vi "twoMPU_alejMarch07.vi"() -> ()   [LabVIEW 2016]
uses:
  <vilib>/MakerHub/LINX/Private/Type Defs/Interface.ctl
  <vilib>/MakerHub/LINX/Public/Sensors/Accelerometer/MPU60X0/Clock Source.ctl
  Control 1.ctl
  <vilib>/MakerHub/LINX/Private/Type Defs/User Platform.ctl
  <vilib>/MakerHub/LINX/Public/Sensors/Accelerometer/MPU60X0/DeviceAddresses.ctl
  <vilib>/MakerHub/LINX/Public/Sensors/Accelerometer/MPU60X0/AccelFullScaleRanges.ctl
  <vilib>/MakerHub/LINX/Public/Sensors/Accelerometer/MPU60X0/GyroFullScaleRanges.ctl
  <vilib>/MakerHub/LINX/Public/Initialize.vi
  <vilib>/express/express shared/transition.llb/Dynamic To Waveform Array.vi
  <vilib>/express/express signal manip/GetorSetDDTAttributes/Set DDT Attributes/SetT0.vi
  <vilib>/express/express shared/transition.llb/Waveform Array To Dynamic.vi
  <vilib>/express/express signal manip/GetorSetDDTAttributes/Set DDT Attributes/Set DDT Properties.xnode
  <vilib>/MakerHub/LINX/LMH-LINX.lvlib
  <vilib>/MakerHub/LINX/Public/Sensors/Accelerometer/MPU60X0/MPU60X0.lvlib
  <vilib>/Platform/NI_3dgraph.lvlib
panel:
  out "Path Length MPU2":dbl
  in  "DATA RECORD":bool
  out "XY Graph 2":cluster{"Y":dbl[], "Y":dbl[]}[](graph)
  in  "Baud Rate Override":T1
  in  "Clock Source 2":T2
  out "Path Length MPU1":dbl
  out "vector error":errorcluster
  in  "Plot of roll and pitch":refnum<k7>(container)
  out "XY Graph":cluster{"Y":dbl[], "Y":dbl[]}[](graph)
  out "error out":errorcluster
  out "MATLAB Error":errorcluster
  out "Error Out":errorcluster
  in  "?":bool
  in  "I2C Channel":u8
  in  "Clock Source":T2
  in  "Interface":T3
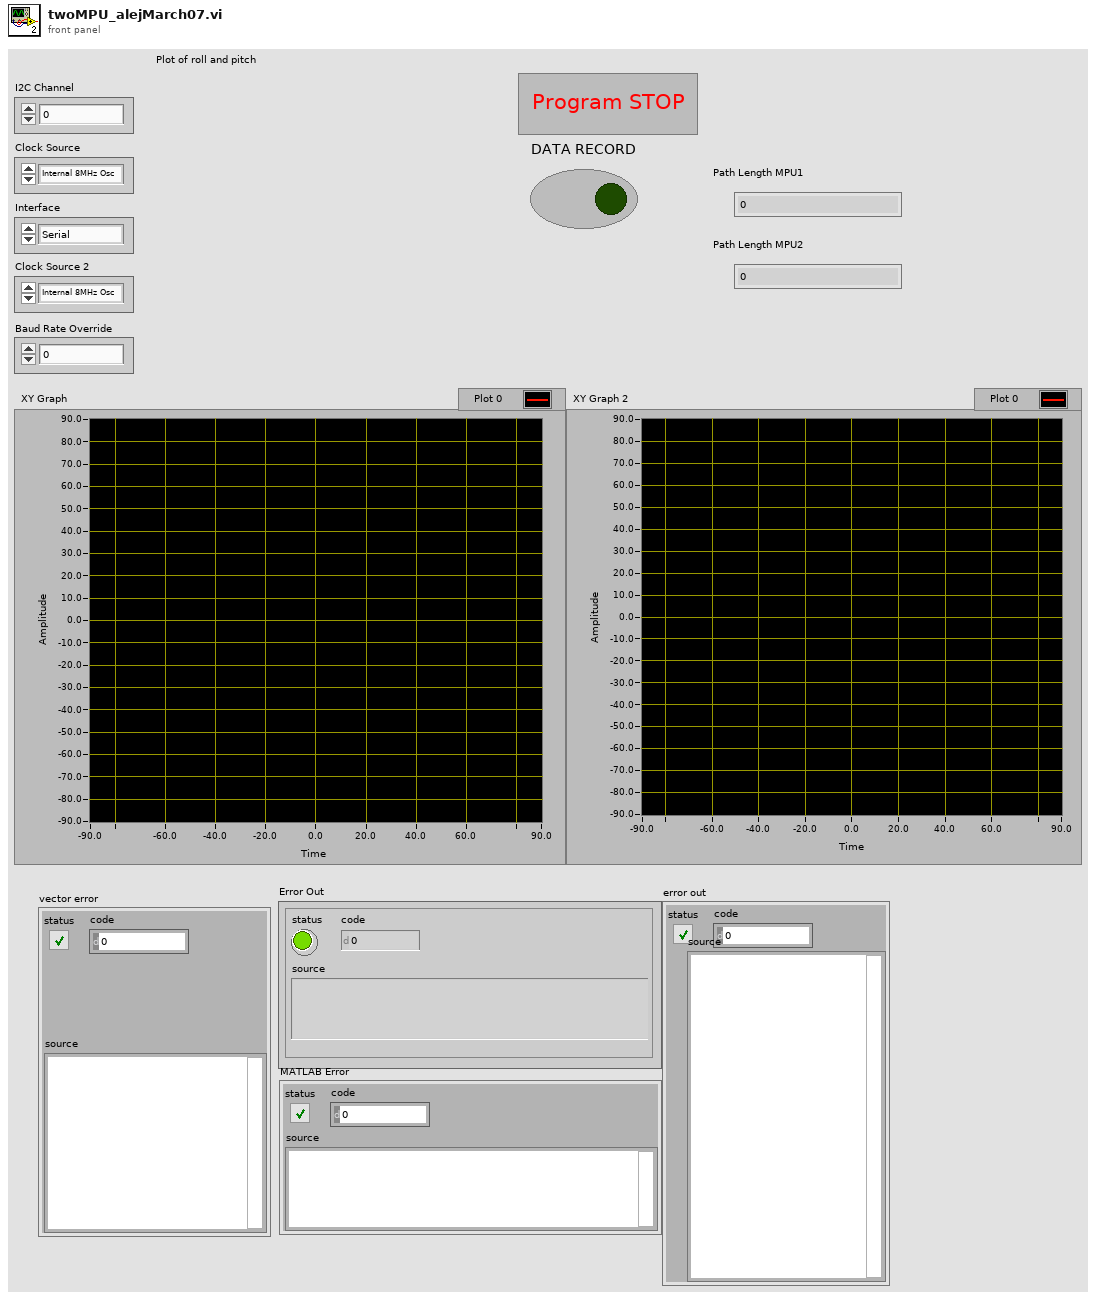
[diagram p1: front panel]
types:
  T1 = typedef "Control 1.ctl" = u32
  T2 = typedef "LMH-LINX.lvlib/MPU60X0.lvlib/Clock Source.ctl" = enum8{"Internal 8MHz Osc", "PLL with X Gyro Ref", "PLL with Y Gyro Ref", "PLL with Z Gyro Ref", "PLL with ext 32.768 KHz Ref", "PLL with ext 19.2 MHz Ref", "Reserved", "Hold in reset"}
  T3 = typedef "LMH-LINX.lvlib/Interface.ctl" = enum16{"Serial", "TCP"}
  T4 = typedef "LMH-LINX.lvlib/MPU60X0.lvlib/DeviceAddresses.ctl" = enum16{"0x68", "0x69"}
  T5 = typedef "LMH-LINX.lvlib/MPU60X0.lvlib/GyroFullScaleRanges.ctl" = enum8{"±250 °/s", "±500 °/s", "±1000 °/s", "±2000 °/s"}
  T6 = typedef "LMH-LINX.lvlib/MPU60X0.lvlib/AccelFullScaleRanges.ctl" = enum16{"±2g", "±4g", "±8g", "±16g"}
  T7 = typedef "LMH-LINX.lvlib/User Platform.ctl" = enum16{"Default", "Remote", "Local"}
  T8 = typedef "LMH-LINX.lvlib/LINX Ref.ctl" = cluster{"IO":T9, "Interface":T3, "LINX Device Config":T10}
  T9 = typedef "LMH-LINX.lvlib/Platform.ctl" = enum16{"Remote", "Local"}
  T10 = typedef "LMH-LINX.lvlib/Device.lvlib/LINX Device Config.ctl" = cluster{"Interface":T3, "COM Port":refnum<visa-resource-name>, "TCP Configuration":T11, "Device Family":u8, "Device ID":u8, "Device Name":string, "TCP Ref":refnum<k5>, "Channels":T12}
  T11 = typedef "LMH-LINX.lvlib/Device.lvlib/TCP Config.ctl" = cluster{"IP Address":string, "Port":u16}
  T12 = typedef "LMH-LINX.lvlib/Channels.ctl" = cluster{"DI":u8[], "DO":u8[], "AI":u8[], "AO":u8[], "PWM":u8[], "QE":u8[], "UART":u8[], "I2C 2":u8[], "SPI":u8[], "CAN":u8[], "Servo":u8[], "AI Ref (V)":dbl, "AI Resolution (Bits)":u8, "AO Ref (V)":dbl, "AO Resolution (Bits)":u8}
  T13 = cluster{"X Axis":i16, "Y Axis":i16, "Z Axis":i16}
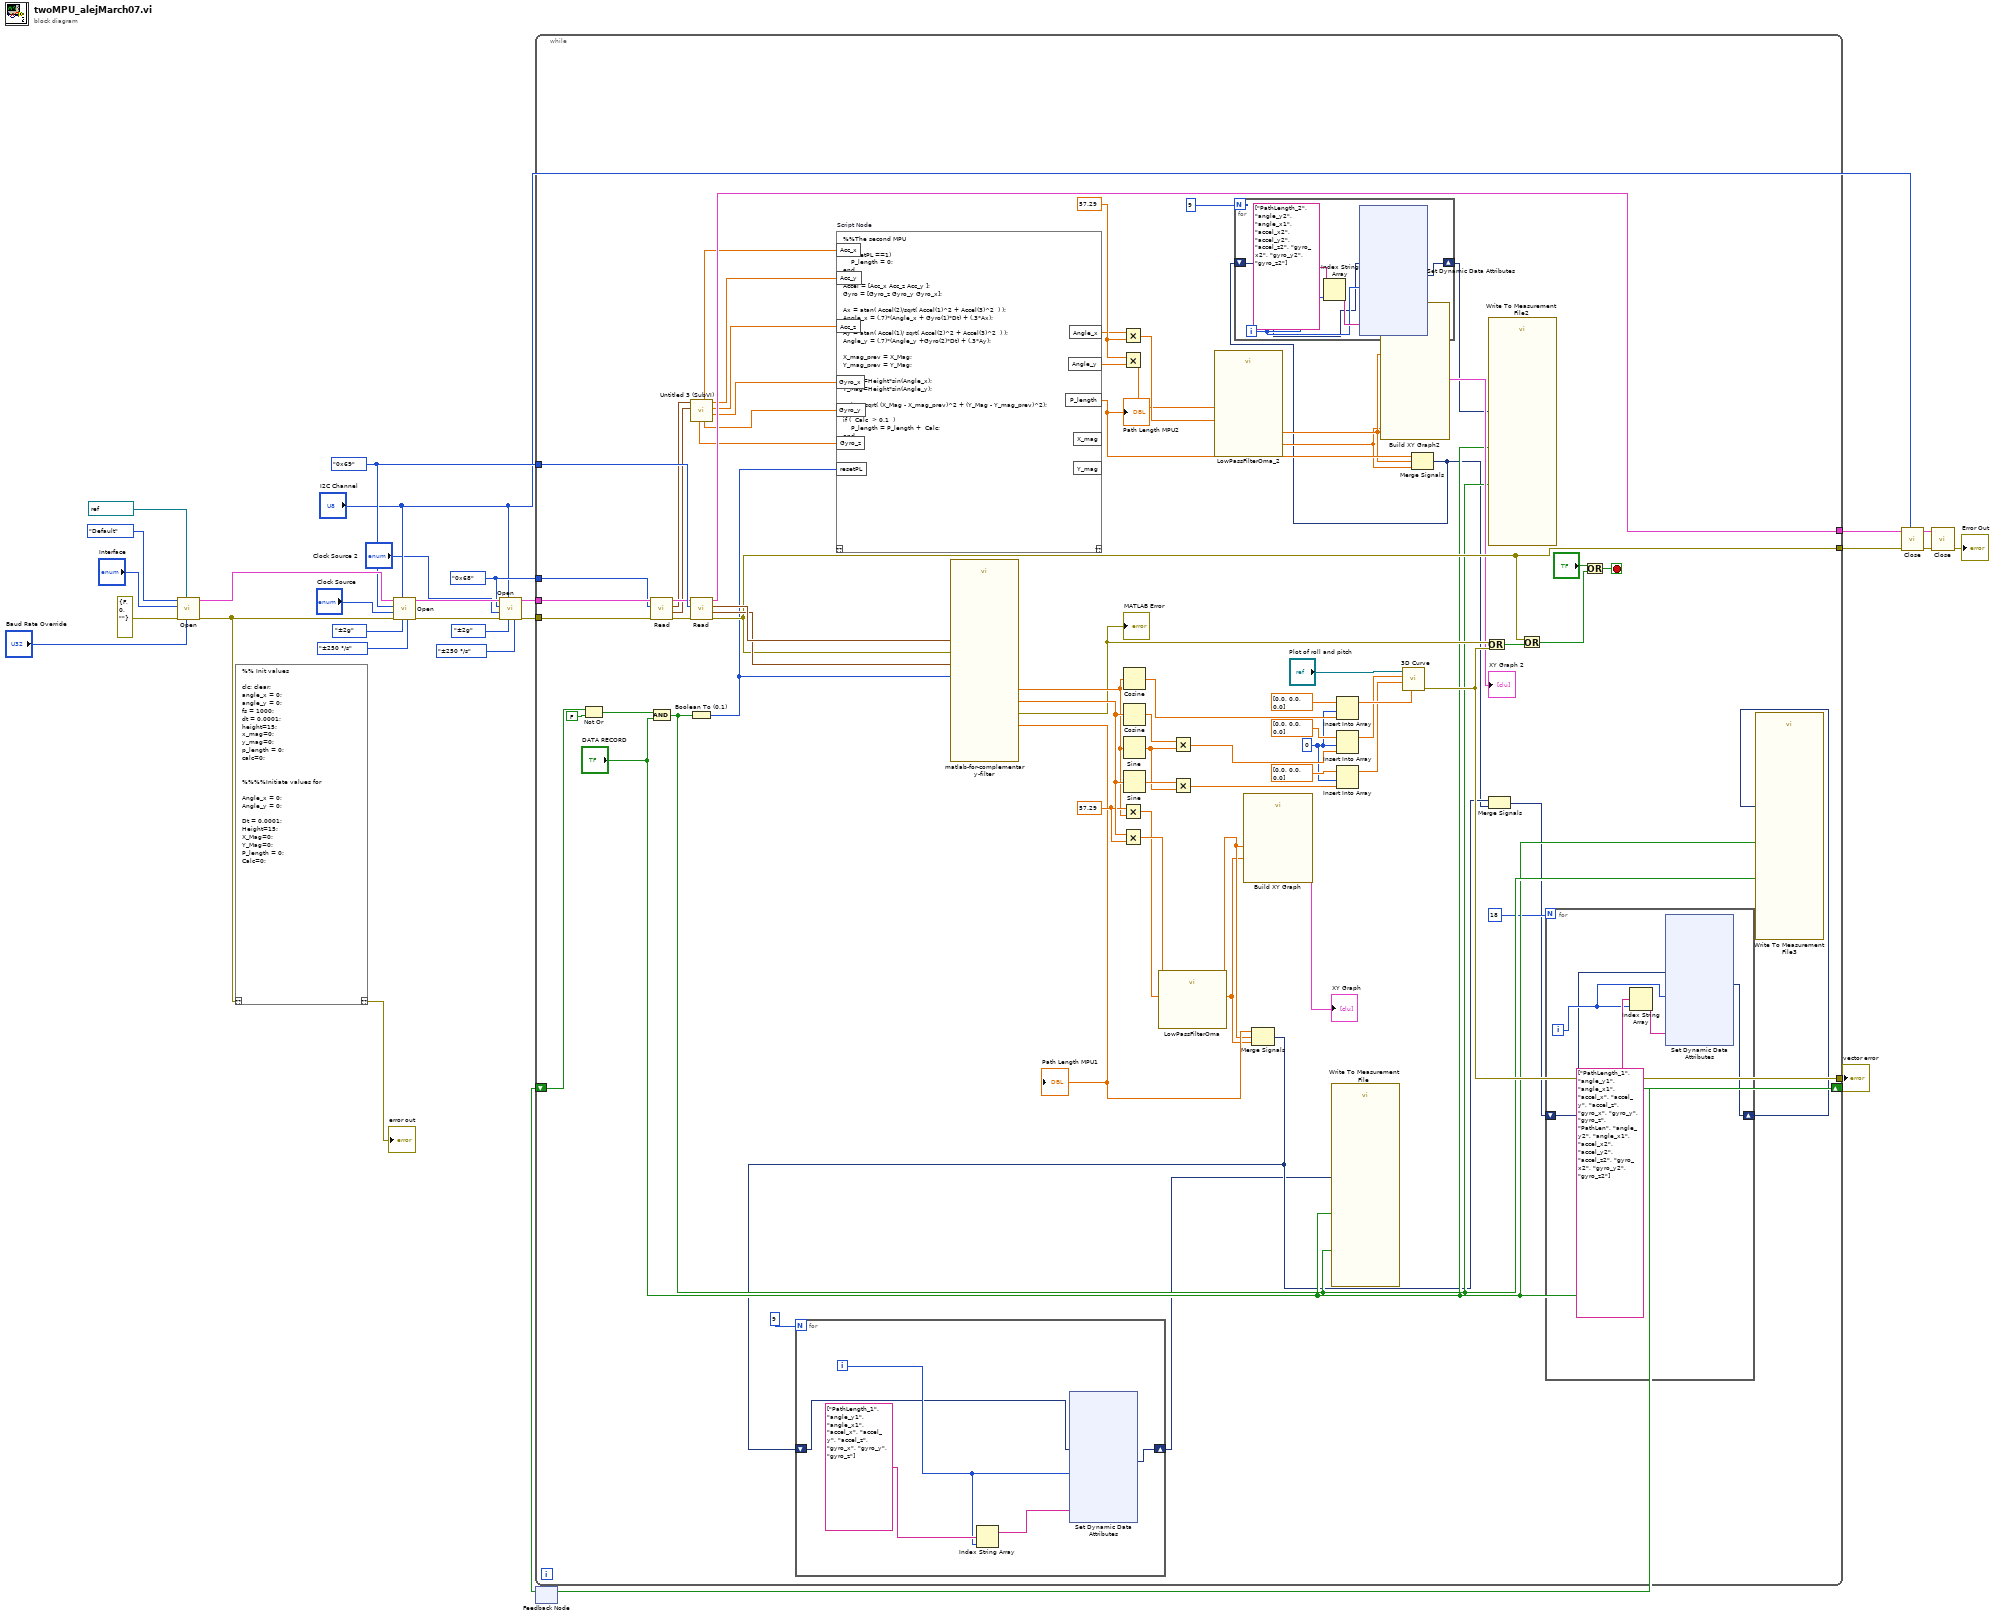
[diagram p0: block diagram]
diagram:
  w7 = DeviceAddresses."0x68" ("I2C Slave Address")
  w24 = DeviceAddresses."0x69" ("Device Address")
  n1 = call-poly <vilib>:"Open.vi"("Baud Rate Override"="Baud Rate Override", "Serial Port"=refnum<visa-resource-name> "COM5", "Error In"=errorcluster {"status"=FALSE, "code"=0, "source"=""}, "Interface"="Interface", "IO"=User_Platform."Default") -> ("Error Out"=w18:errorcluster, "LINX Resource"=w27:T8)  [unwired: 4 in, 1 out]
  n2 = script code="%% Init values\n\nclc; clear;\nangle_x = 0;\nangle_y = 0;\nfs = 1000;\ndt = 0.0001;\nheight=15;\nx_mag=0; \ny_mag=0; \np_length = 0;\ncalc=0;\n\n\n%%%%Initiate values for \n\nAngle_x = 0;\nAngle_y = 0;\n\nDt = 0.0001;\nHeight=15;\nX_Mag=0; \nY_Mag=0; \nP_length = 0;\nCalc=0;"("??"=w18) -> ("??"=→"error out":errorcluster)
  n3 = call <vilib>:"Open.vi"("Gyro Full Scale Range"=GyroFullScaleRanges."±250 °/s", "Accel Full Scale Range"=AccelFullScaleRanges."±2g", "I2C Channel"="I2C Channel", "Error In"=w18, "Clock Source"="Clock Source", "I2C Slave Address"=w24, "LINX Resource"=w27) -> ("Error Out"=w9:errorcluster, "LINX Resource"=w13:T8)  [unwired: 3 in]
  n4 = call <vilib>:"Open.vi"("Gyro Full Scale Range"=GyroFullScaleRanges."±250 °/s", "Accel Full Scale Range"=AccelFullScaleRanges."±2g", "I2C Channel"="I2C Channel", "Error In"=w9, "Clock Source"="Clock Source 2", "I2C Slave Address"=w7, "LINX Resource"=w13) -> ("Error Out"=w8:errorcluster, "LINX Resource"=w12:T8)  [unwired: 3 in]
  n5 = feedback #1() -> (w1:bool)  [unwired: 1 in]
  n6 = while {
    tunnel: w12 -> [w72]
    tunnel: w24 -> [w100]
    tunnel: [w99] -> w23
    tunnel: [w75] -> w21
    tunnel: [w76] -> w14
    tunnel: w8 -> [w69]
    tunnel: w7 -> [w70]
    shift-right: ["DATA RECORD"] -> w2
    shift-left: w1 -> [w50]
    stop <- w79 stop-if-true
    w60 = 57.29 ("y")
    w83 = 57.29 ("y")
    w85 = 0 ("index")
    n7 = Not Or(1:FALSE ("y"), 2:w50) -> (0:w48:bool)
    n8 = call <vilib>:"Read.vi"("Error In"=w69, "I2C Slave Address"=w70, "LINX Resource"=w72) -> ("Error Out"=w68:errorcluster, "Gyro  Data (dps)"=w61:T13, "Acceleration Data (g)"=w62:T13, "LINX Resource"=w71:T8)  [unwired: 4 in, 1 out]
    n9 = And(x=w48, y="DATA RECORD") -> (x .and. y?=w47:bool)
    n10 = call "Untitled 3 (SubVI).vi"("Gyro  Data (dps)"=w61, "Acceleration Data (g)"=w62) -> ("Gyro_X"=w32:dbl, "Accel_Z"=w33:dbl, "Accel_Y"=w34:dbl, "Gyro_Y"=w31:dbl, "Accel_X"=w35:dbl, "Gyro_Z"=w30:dbl)  [unwired: 4 in]
    n11 = call <vilib>:"Read.vi"("Error In"=w68, "I2C Slave Address"=w100, "LINX Resource"=w71) -> ("Error Out"=w75:errorcluster, "Gyro  Data (dps)"=w97:T13, "Acceleration Data (g)"=w98:T13, "LINX Resource"=w99:T8)  [unwired: 4 in, 1 out]
    n12 = Boolean To (0,1)(Boolean=w47) -> (0, 1=w45:i16)
    n13 = script code="%%The second MPU \n\nif (resetPL ==1) \n    P_length = 0;\nend\n\nAccel = [Acc_x Acc_z Acc_y ];\nGyro = [Gyro_z Gyro_y Gyro_x];\n\nAx = atan( Accel(2)/sqrt( Accel(1)^2 + Accel(3)^2  ) );\nAngle_x = (.7)*(Angle_x + Gyro(1)*Dt) + (.3*Ax);\n\nAy = atan( Accel(1)/ sqrt( Accel(2)^2 + Accel(3)^2  ) );\nAngle_y = (.7)*(Angle_y +Gyro(2)*Dt) + (.3*Ay);\n\nX_mag_prev = X_Mag;\nY_mag_prev = Y_Mag;\n\nX_Mag=Height*sin(Angle_x); \nY_Mag=Height*sin(Angle_y);\n\nCalc = sqrt( (X_Mag - X_mag_prev)^2 + (Y_Mag - Y_mag_prev)^2);\n\nif (  Calc  > 0.1  ) \n    P_length = P_length +  Calc;\nend" "Script Node"("Acc_x"=w35, "Acc_y"=w34, "Acc_z"=w33, "Gyro_x"=w32, "Gyro_y"=w31, "Gyro_z"=w30, "resetPL"=w45) -> ("Angle_x"=w59:dbl, "Angle_y"=w58:dbl, "P_length"=w55:dbl)  [unwired: 1 in, 3 out]
    "Path Length MPU2" <- w55
    n14 = call "matlab-for-complementary-filter.vi"("Acceleration Data (g)"=w98, "Gyro  Data (dps)"=w97, "PLRESET"=w45, "error in (no error)"=w75) -> ("angle_y"=w84:dbl, "Path Length"=w65:dbl, "angle_x"=w82:dbl, "error out"=w77:errorcluster)  [unwired: 10 in, 2 out]
    "MATLAB Error" <- w77
    "Path Length MPU1" <- w65
    n15 = Multiply(x=w59, y=w60) -> (x*y=w54:dbl)
    n16 = Multiply(x=w60, y=w58) -> (x*y=w53:dbl)
    n17 = Multiply(x=w83, y=w82) -> (x*y=w66:dbl)
    n18 = Multiply(x=w84, y=w83) -> (x*y=w67:dbl)
    n19 = Cosine(x=w82) -> (cos(x)=w87:dbl)
    n20 = Cosine(x=w84) -> (cos(x)=w96:dbl)
    n21 = Sine(x=w82) -> (sin(x)=w90:dbl)
    n22 = Sine(x=w84) -> (sin(x)=w91:dbl)
    n23 = call "LowPassFilterOma.vi"("Numeric"=w66, "Numeric 2"=w67) -> ("Filtered x"=w63:dbl, "Filtered x 2"=w64:dbl)  [unwired: 8 in]
    n24 = Multiply(x=w96, y=w90) -> (x*y=w93:dbl)
    n25 = Multiply(x=w91, y=w90) -> (x*y=w89:dbl)
    n26 = call "LowPassFilterOma_2.vi"("Angle_y_2"=w53, "Angle_x_2"=w54) -> ("y_filt_2"=w51:dbl, "x_filt_2"=w52:dbl)  [unwired: 8 in]
    n27 = call "Build XY Graph"("Y Input"=w63, "X Input"=w64) -> ("XY Graph"=→"XY Graph":cluster{"X":dbl[], "Y":dbl[]}[])  [unwired: 8 in, 1 out]
    n28 = Merge Signals(w65, w64, w63) -> (w43:dynamicdata)
    n29 = for {
      N: 9 -> [_]
      shift-right: [w137] -> w42
      shift-left: w43 -> [w138]
      i -> [w139]
      n30 = Index String Array(1:w139, 2:string[] ["PathLength_1", "angle_y1", "angle_x1", "accel_x", "accel_y", "accel_z", "gyro_x", "gyro_y", "gyro_z"]) -> (0:w140:string)  [unwired: 1 in]
      n31 = xnode "Set Dynamic Data Attributes"("Signals In"=w138, "Signal Index"=w139, "Signal Name"=w140) -> ("Signals Out"=w137:dynamicdata)  [unwired: 1 in, 1 out]
    }
    n32 = call "Write To Measurement File"("Signals"=w42, "Enable"="DATA RECORD", "new_file"=w47) -> ()  [unwired: 14 in, 3 out]
    n33 = Insert Into Array(array=dbl[] [0.0, 0.0, 0.0], index=w85, new element=w87) -> (w86:dbl[])
    n34 = Insert Into Array(array=dbl[] [0.0, 0.0, 0.0], index=w85, new element=w93) -> (w81:dbl[])
    n35 = Insert Into Array(array=dbl[] [0.0, 0.0, 0.0], index=w85, new element=w89) -> (w80:dbl[])
    n36 = call "Build XY Graph2"("Y Input"=w51, "X Input"=w52) -> ("XY Graph"=→"XY Graph 2":cluster{"X":dbl[], "Y":dbl[]}[])  [unwired: 8 in, 1 out]
    n37 = call <vilib>:"3D Curve.vi"("z vector"=w86, "y vector"=w80, "x vector"=w81, "3D graph"="Plot of roll and pitch") -> ("error out"=w76:errorcluster)  [unwired: 6 in, 1 out]
    n38 = Merge Signals(w55, w52, w51) -> (w39:dynamicdata)
    n39 = for {
      N: 9 -> [_]
      shift-right: [w102] -> w38
      shift-left: w39 -> [w101]
      i -> [w103]
      n40 = Index String Array(1:w103, 2:string[] ["PathLength_2", "angle_y2", "angle_x1", "accel_x2", "accel_y2", "accel_z2", "gyro_x2", "gyro_y2", "gyro_z2"]) -> (0:w104:string)  [unwired: 1 in]
      n41 = xnode "Set Dynamic Data Attributes"("Signals In"=w101, "Signal Index"=w103, "Signal Name"=w104) -> ("Signals Out"=w102:dynamicdata)  [unwired: 1 in, 1 out]
    }
    n42 = Or(x=w77, y=w76) -> (x .or. y?=w78:bool)
    n43 = call "Write To Measurement File2"("Signals"=w38, "Enable"="DATA RECORD", "new_file"=w47) -> ()  [unwired: 14 in, 3 out]
    n44 = Merge Signals(w43, w39) -> (w37:dynamicdata)
    n45 = Or(x=w75, y=w78) -> (x .or. y?=w73:bool)
    n46 = for {
      N: 18 -> [_]
      shift-right: [w119] -> w36
      shift-left: w37 -> [w120]
      i -> [w121]
      n47 = Index String Array(1:w121, 2:string[] ["PathLength_1", "angle_y1", "angle_x1", "accel_x", "accel_y", "accel_z", "gyro_x", "gyro_y", "gyro_z", "PathLen", "angle_y2", "angle_x1", "accel_x2", "accel_y2", "accel_z2", "gyro_x2", "gyro_y2", "gyro_z2"]) -> (0:w123:string)  [unwired: 1 in]
      n48 = xnode "Set Dynamic Data Attributes"("Signals In"=w120, "Signal Index"=w121, "Signal Name"=w123) -> ("Signals Out"=w119:dynamicdata)  [unwired: 1 in, 1 out]
    }
    n49 = Or(x="?", y=w73) -> (x .or. y?=w79:bool)
    n50 = call "Write To Measurement File3"("Signals"=w36, "Enable"="DATA RECORD", "new_file"=w47) -> ()  [unwired: 14 in, 3 out]
  }
  "vector error" <- w14
  n51 = feedback-in #1(w2) -> ()
  n52 = call <vilib>:"Close.vi"("I2C Channel (0)"="I2C Channel", "Error In"=w21, "LINX Resource"=w23) -> ("Error Out"=w20:errorcluster, "LINX Resource"=w22:T8)  [unwired: 7 in]
  n53 = call <vilib>:"Close.vi"("Error In"=w20, "LINX Resource"=w22) -> ("Error Out"=→"Error Out":errorcluster)  [unwired: 9 in]
